vi "Joystick_Test.vi"(9 "input cluster":T7) -> (2 "RobotDriveDevRef":T1={"DevStatus"={"status"=FALSE, "code"=0, "source"=""}, "Motors[]"=[], "Square Inputs"=FALSE, "Max Output"=1.0})   [LabVIEW 2020]
uses:
  <vilib>/Rock Robotics/WPI/RobotDrive/WPI_RobotDriveDevRef.ctl
  <vilib>/Rock Robotics/WPI/MotorControl/WPI_MotorControlDeviceRef.ctl
  <vilib>/Rock Robotics/WPI/MotorControl/WPI_MotorControlType.ctl
  <vilib>/Rock Robotics/SystemInterfaces/DIO/FPGA_DIOPWMChannel.ctl
  <vilib>/Rock Robotics/WPI/PWM/WPI_PWMDeadband.ctl
  <vilib>/Rock Robotics/SystemInterfaces/DIO/FPGA_DIOChannel.ctl
  <vilib>/Rock Robotics/WPI/Utilities/WPI_GetSetVariantRefNum.vi
  <vilib>/Rock Robotics/Network Tables/NT Write Number.vi
  GlobalVariables.vi
  <vilib>/Rock Robotics/WPI/RobotDrive/WPI_RobotDriveArcadeDrive_Standard(NoSaturation).vi
  <vilib>/Rock Robotics/WPI/ThirdParty/Phoenix-LabVIEW/Motor Controller/Controls/CTRE_Phoenix_MotorControl_ControlMode.ctl
panel:
  out "L_X":dbl
  out "L_Y":dbl
  out "Axes[3]":dbl
  out "Axes[2]":dbl
  out "Motor Values":dbl[](array[numeric])
  out "Axes[1]":dbl
  out "Axes[0]":dbl
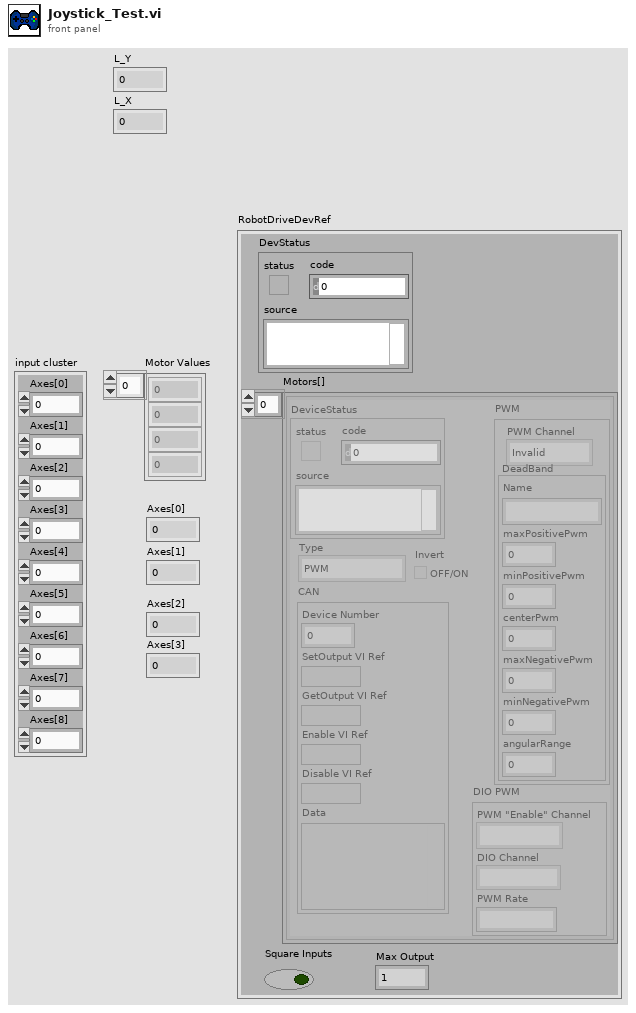
[diagram p1: front panel]
types:
  T1 = typedef "WPI_RobotDriveDevRef.ctl" = cluster{"DevStatus":errorcluster, "Motors[]":T2[], "Square Inputs":bool, "Max Output":dbl}
  T2 = typedef "WPI_MotorControlDeviceRef.ctl" = cluster{"DeviceStatus":errorcluster, "Type":T3, "PWM":cluster{"PWM Channel":T4, "DeadBand":T5}, "CAN":cluster{"Device Number":u8, "SetOutput VI Ref":variant, "GetOutput VI Ref":variant, "Enable VI Ref":variant, "Disable VI Ref":variant, "Data":variant}, "Invert":bool, "DIO PWM":cluster{"PWM \"Enable\" Channel":T4, "DIOChannel":T6, "PWM Rate":dbl}}
  T3 = typedef "WPI_MotorControlType.ctl" = enum16{"PWM", "CAN", "DIO PWM"}
  T4 = typedef "FPGA_DIOPWMChannel.ctl" = enum8{"PWM 0", "PWM 1", "PWM 2", "PWM 3", "PWM 4", "PWM 5", "PWM 6", "PWM 7", "PWM 8", "PWM 9", "PWM MXP 0", "PWM MXP 1", "PWM MXP 2", "PWM MXP 3", "PWM MXP 4", "PWM MXP 5", "PWM MXP 6", "PWM MXP 7", "PWM MXP 8", "PWM MXP 9", "Invalid"}
  T5 = typedef "WPI_PWMDeadband.ctl" = cluster{"Name":string, "maxPositivePwm":i32, "minPositivePwm":i32, "centerPwm":i32, "maxNegativePwm":i32, "minNegativePwm":i32, "angularRange":u16}
  T6 = typedef "FPGA_DIOChannel.ctl" = enum8{"DIO 0", "DIO 1", "DIO 2", "DIO 3", "DIO 4", "DIO 5", "DIO 6", "DIO 7", "DIO 8", "DIO 9", "DIO MXP 0", "DIO MXP 1", "DIO MXP 2", "DIO MXP 3", "DIO MXP 4", "DIO MXP 5", "DIO MXP 6", "DIO MXP 7", "DIO MXP 8", "DIO MXP 9", "DIO MXP 10", "DIO MXP 11", "DIO MXP 12", "DIO MXP 13", "DIO MXP 14", "DIO MXP 15", "SPI Port CS1", "SPI Port CS2", "SPI Port CS3", "SPI Port MISO", "SPI Port MOSI", "Invalid"}
  T7 = cluster{"Axes[0]":dbl, "Axes[1]":dbl, "Axes[2]":dbl, "Axes[3]":dbl, "Axes[4]":dbl, "Axes[5]":dbl, "Axes[6]":dbl, "Axes[7]":dbl, "Axes[8]":dbl}
  T8 = typedef "CTRE_Phoenix_MotorControl_ControlMode.ctl" = u16
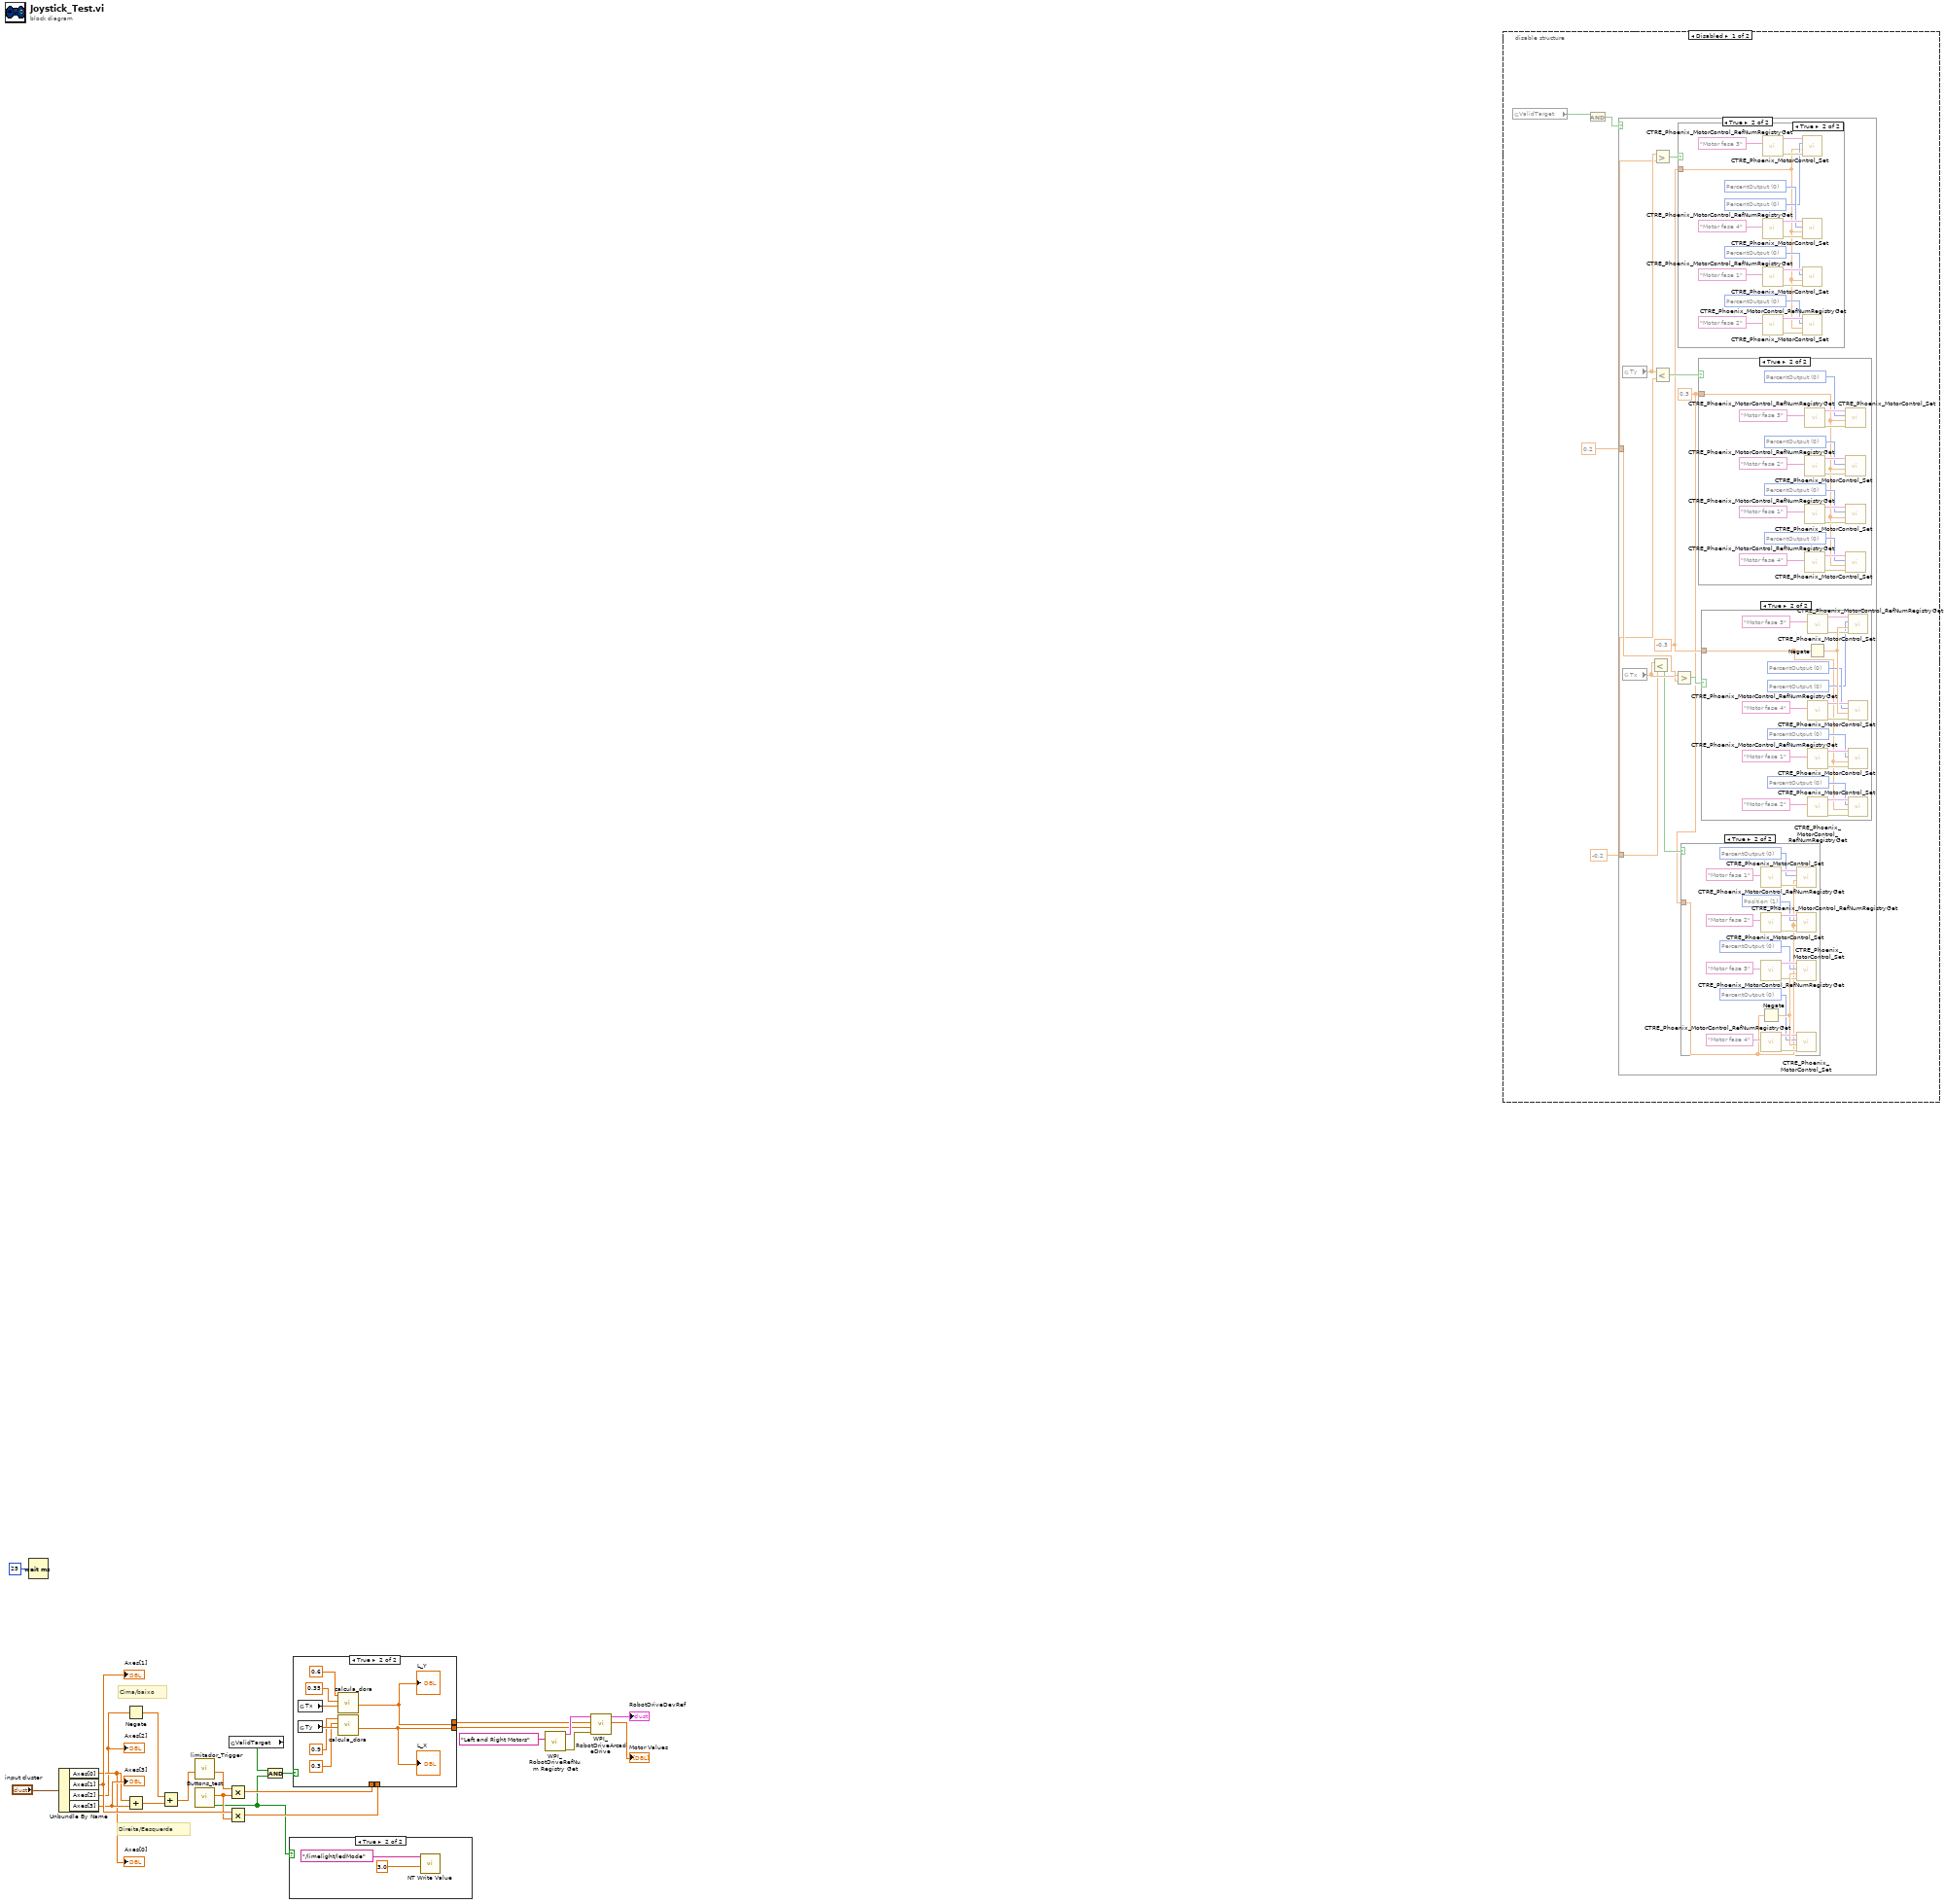
[diagram p0: block diagram]
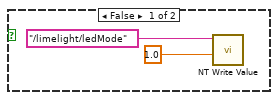
[diagram p2: hidden frame]
diagram:
  # "Direita/Eesquerda"
  # "Cima/baixo"
  n1 = Wait (ms)(milliseconds to wait=u32 25) -> ()  [unwired: 1 out]
  n2 = Unbundle By Name("input cluster") -> ("Axes[0]"=w19:dbl, "Axes[1]"=w23:dbl, "Axes[2]"=w16:dbl, "Axes[3]"=w21:dbl)
  "Axes[0]" <- w19
  "Axes[1]" <- w23
  "Axes[2]" <- w16
  "Axes[3]" <- w21
  n3 = Negate(x=w16) -> (-x=w15:dbl)
  n4 = Add(x=w19, y=w21) -> (x+y=w20:dbl)
  n5 = Add(x=w15, y=w20) -> (x+y=w18:dbl)
  n6 = call "limitador_Trigger.vi"("IN"=w18) -> ("OUT"=w17:dbl)  [unwired: 10 in]
  n7 = call "Buttons_test.vi"() -> ("Buttons[6]"=w1:bool, "OUT"=w22:dbl)  [unwired: 8 in]
  n8 = Multiply(x=w17, y=w22) -> (x*y=w4:dbl)
  n9 = Multiply(x=w23, y=w22) -> (x*y=w5:dbl)
  n10 = global read "GlobalVariables.vi" "ValidTarget"() -> (w11:bool)
  n11 = And(x=w11, y=w1) -> (x .and. y?=w12:bool)
  n12 = case shown="True" w1 {
    frame False {
      n13 = call-poly <vilib>:"NT Write Value.vi"("Numeric"=1.0, "Name"="/limelight/ledMode") -> ()  [unwired: 9 in, 1 out]
    }
    frame True {
      n14 = call-poly <vilib>:"NT Write Value.vi"("Numeric"=3.0, "Name"="/limelight/ledMode") -> ()  [unwired: 9 in, 1 out]
    }
  }
  n15 = case shown="True" w12 {
    tunnel: w5 -> [w29 _]
    tunnel: w4 -> [w28 _]
    tunnel: [w29 w34] -> w3
    tunnel: [w28 w37] -> w2
    frame False {
    }
    frame True {
      n16 = global read "GlobalVariables.vi" "Tx"() -> (w36:dbl)
      n17 = global read "GlobalVariables.vi" "Ty"() -> (w35:dbl)
      n18 = call "calcula_dora.vi"("x"=w36, "Mot_Min"=0.35, "Mot_Max"=0.6) -> ("x+y"=w37:dbl)  [unwired: 8 in]
      "L_Y" <- w37
      n19 = call "calcula_dora.vi"("x"=w35, "Mot_Min"=0.3, "Mot_Max"=0.9) -> ("x+y"=w34:dbl)  [unwired: 8 in]
      "L_X" <- w34
    }
  }
  n20 = call <vilib>:"WPI_RobotDriveRefNum Registry Get.vi"("refnum name"="Left and Right Motors") -> ("error out"=w7:errorcluster, "RobotDriveDevRef"=w9:T1)  [unwired: 9 in]
  n21 = call-poly <vilib>:"WPI_RobotDriveArcadeDrive.vi"("error in (no error)"=w7, "Y axis value"=w3, "X axis value"=w2, "RobotDriveDevRef"=w9) -> ("Motor Values"=→"Motor Values":dbl[], "RobotDriveDevRef"=→"RobotDriveDevRef":T1)  [unwired: 5 in, 1 out]
  n22 = disable-structure shown="Disabled" {
    frame Disabled {
      n23 = global read "GlobalVariables.vi" "ValidTarget"() -> (w41:bool)
      n24 = And(x=w41) -> (x .and. y?=w40:bool)  [unwired: 1 in]
      n25 = case shown="True" w40 {
        tunnel: 0.2 -> [_ w45]
        tunnel: -0.2 -> [_ w44]
        frame False {
        }
        frame True {
          w42 = 0.3
          w43 = -0.3
          n26 = global read "GlobalVariables.vi" "Ty"() -> (w47:dbl)
          n27 = global read "GlobalVariables.vi" "Tx"() -> (w50:dbl)
          n28 = Less?(x=w50, y=w44) -> (x < y?=w49:bool)
          n29 = Greater?(x=w47, y=w45) -> (0:w48:bool)
          n30 = Less?(x=w47, y=w44) -> (x < y?=w46:bool)
          n31 = Greater?(x=w50, y=w45) -> (0:w51:bool)
          n32 = case shown="True" w48 {
            tunnel: w43 -> [_ w69]
            frame False {
            }
            frame True {
              w77 = T8 0 items=["PercentOutput"=0, "Position"=1, "Velocity"=2, "Current"=3, "Follower"=5, "MotionProfile"=6, "MotionMagic"=7, "MotionProfileArc"=10, "Disabled"=15] ("Control Mode")
              w75 = T8 0 items=["PercentOutput"=0, "Position"=1, "Velocity"=2, "Current"=3, "Follower"=5, "MotionProfile"=6, "MotionMagic"=7, "MotionProfileArc"=10, "Disabled"=15] ("Control Mode")
              w73 = T8 0 items=["PercentOutput"=0, "Position"=1, "Velocity"=2, "Current"=3, "Follower"=5, "MotionProfile"=6, "MotionMagic"=7, "MotionProfileArc"=10, "Disabled"=15] ("Control Mode")
              w71 = T8 0 items=["PercentOutput"=0, "Position"=1, "Velocity"=2, "Current"=3, "Follower"=5, "MotionProfile"=6, "MotionMagic"=7, "MotionProfileArc"=10, "Disabled"=15] ("Control Mode")
              n33 = call <vilib>:"CTRE_Phoenix_MotorControl_RefNumRegistryGet.vi"("refnum name"="Motor fase 3") -> ("error out"=w79:errorcluster, "PhoenixMotorControlDevRef"=w78:T2)  [unwired: 9 in]
              n34 = call <vilib>:"CTRE_Phoenix_MotorControl_RefNumRegistryGet.vi"("refnum name"="Motor fase 4") -> ("error out"=w81:errorcluster, "PhoenixMotorControlDevRef"=w80:T2)  [unwired: 9 in]
              n35 = call <vilib>:"CTRE_Phoenix_MotorControl_RefNumRegistryGet.vi"("refnum name"="Motor fase 1") -> ("error out"=w83:errorcluster, "PhoenixMotorControlDevRef"=w82:T2)  [unwired: 9 in]
              n36 = call <vilib>:"CTRE_Phoenix_MotorControl_RefNumRegistryGet.vi"("refnum name"="Motor fase 2") -> ("error out"=w85:errorcluster, "PhoenixMotorControlDevRef"=w84:T2)  [unwired: 9 in]
              n37 = call <vilib>:"CTRE_Phoenix_MotorControl_Set.vi"("error in (no error)"=w79, "Output"=w69, "Control Mode"=w71, "PhoenixMotorControlDevRef"=w78) -> ()  [unwired: 6 in, 2 out]
              n38 = call <vilib>:"CTRE_Phoenix_MotorControl_Set.vi"("error in (no error)"=w81, "Output"=w69, "Control Mode"=w73, "PhoenixMotorControlDevRef"=w80) -> ()  [unwired: 6 in, 2 out]
              n39 = call <vilib>:"CTRE_Phoenix_MotorControl_Set.vi"("error in (no error)"=w83, "Output"=w69, "Control Mode"=w75, "PhoenixMotorControlDevRef"=w82) -> ()  [unwired: 6 in, 2 out]
              n40 = call <vilib>:"CTRE_Phoenix_MotorControl_Set.vi"("error in (no error)"=w85, "Output"=w69, "Control Mode"=w77, "PhoenixMotorControlDevRef"=w84) -> ()  [unwired: 6 in, 2 out]
            }
          }
          n41 = case shown="True" w49 {
            tunnel: w42 -> [_ w86]
            frame False {
            }
            frame True {
              w94 = T8 0 items=["PercentOutput"=0, "Position"=1, "Velocity"=2, "Current"=3, "Follower"=5, "MotionProfile"=6, "MotionMagic"=7, "MotionProfileArc"=10, "Disabled"=15] ("Control Mode")
              w92 = T8 0 items=["PercentOutput"=0, "Position"=1, "Velocity"=2, "Current"=3, "Follower"=5, "MotionProfile"=6, "MotionMagic"=7, "MotionProfileArc"=10, "Disabled"=15] ("Control Mode")
              w90 = T8 1 items=["PercentOutput"=0, "Position"=1, "Velocity"=2, "Current"=3, "Follower"=5, "MotionProfile"=6, "MotionMagic"=7, "MotionProfileArc"=10, "Disabled"=15] ("Control Mode")
              w88 = T8 0 items=["PercentOutput"=0, "Position"=1, "Velocity"=2, "Current"=3, "Follower"=5, "MotionProfile"=6, "MotionMagic"=7, "MotionProfileArc"=10, "Disabled"=15] ("Control Mode")
              n42 = call <vilib>:"CTRE_Phoenix_MotorControl_RefNumRegistryGet.vi"("refnum name"="Motor fase 1") -> ("error out"=w96:errorcluster, "PhoenixMotorControlDevRef"=w95:T2)  [unwired: 9 in]
              n43 = call <vilib>:"CTRE_Phoenix_MotorControl_RefNumRegistryGet.vi"("refnum name"="Motor fase 2") -> ("error out"=w98:errorcluster, "PhoenixMotorControlDevRef"=w97:T2)  [unwired: 9 in]
              n44 = call <vilib>:"CTRE_Phoenix_MotorControl_RefNumRegistryGet.vi"("refnum name"="Motor fase 3") -> ("error out"=w100:errorcluster, "PhoenixMotorControlDevRef"=w99:T2)  [unwired: 9 in]
              n45 = Negate(x=w86) -> (-x=w103:dbl)
              n46 = call <vilib>:"CTRE_Phoenix_MotorControl_RefNumRegistryGet.vi"("refnum name"="Motor fase 4") -> ("error out"=w102:errorcluster, "PhoenixMotorControlDevRef"=w101:T2)  [unwired: 9 in]
              n47 = call <vilib>:"CTRE_Phoenix_MotorControl_Set.vi"("error in (no error)"=w96, "Output"=w86, "Control Mode"=w88, "PhoenixMotorControlDevRef"=w95) -> ()  [unwired: 6 in, 2 out]
              n48 = call <vilib>:"CTRE_Phoenix_MotorControl_Set.vi"("error in (no error)"=w98, "Output"=w86, "Control Mode"=w90, "PhoenixMotorControlDevRef"=w97) -> ()  [unwired: 6 in, 2 out]
              n49 = call <vilib>:"CTRE_Phoenix_MotorControl_Set.vi"("error in (no error)"=w100, "Output"=w103, "Control Mode"=w92, "PhoenixMotorControlDevRef"=w99) -> ()  [unwired: 6 in, 2 out]
              n50 = call <vilib>:"CTRE_Phoenix_MotorControl_Set.vi"("error in (no error)"=w102, "Output"=w103, "Control Mode"=w94, "PhoenixMotorControlDevRef"=w101) -> ()  [unwired: 6 in, 2 out]
            }
          }
          n51 = case shown="True" w46 {
            tunnel: w42 -> [_ w52]
            frame False {
            }
            frame True {
              w60 = T8 0 items=["PercentOutput"=0, "Position"=1, "Velocity"=2, "Current"=3, "Follower"=5, "MotionProfile"=6, "MotionMagic"=7, "MotionProfileArc"=10, "Disabled"=15] ("Control Mode")
              w58 = T8 0 items=["PercentOutput"=0, "Position"=1, "Velocity"=2, "Current"=3, "Follower"=5, "MotionProfile"=6, "MotionMagic"=7, "MotionProfileArc"=10, "Disabled"=15] ("Control Mode")
              w56 = T8 0 items=["PercentOutput"=0, "Position"=1, "Velocity"=2, "Current"=3, "Follower"=5, "MotionProfile"=6, "MotionMagic"=7, "MotionProfileArc"=10, "Disabled"=15] ("Control Mode")
              w54 = T8 0 items=["PercentOutput"=0, "Position"=1, "Velocity"=2, "Current"=3, "Follower"=5, "MotionProfile"=6, "MotionMagic"=7, "MotionProfileArc"=10, "Disabled"=15] ("Control Mode")
              n52 = call <vilib>:"CTRE_Phoenix_MotorControl_RefNumRegistryGet.vi"("refnum name"="Motor fase 3") -> ("error out"=w62:errorcluster, "PhoenixMotorControlDevRef"=w61:T2)  [unwired: 9 in]
              n53 = call <vilib>:"CTRE_Phoenix_MotorControl_RefNumRegistryGet.vi"("refnum name"="Motor fase 2") -> ("error out"=w68:errorcluster, "PhoenixMotorControlDevRef"=w67:T2)  [unwired: 9 in]
              n54 = call <vilib>:"CTRE_Phoenix_MotorControl_RefNumRegistryGet.vi"("refnum name"="Motor fase 1") -> ("error out"=w66:errorcluster, "PhoenixMotorControlDevRef"=w65:T2)  [unwired: 9 in]
              n55 = call <vilib>:"CTRE_Phoenix_MotorControl_RefNumRegistryGet.vi"("refnum name"="Motor fase 4") -> ("error out"=w64:errorcluster, "PhoenixMotorControlDevRef"=w63:T2)  [unwired: 9 in]
              n56 = call <vilib>:"CTRE_Phoenix_MotorControl_Set.vi"("error in (no error)"=w62, "Output"=w52, "Control Mode"=w54, "PhoenixMotorControlDevRef"=w61) -> ()  [unwired: 6 in, 2 out]
              n57 = call <vilib>:"CTRE_Phoenix_MotorControl_Set.vi"("error in (no error)"=w68, "Output"=w52, "Control Mode"=w60, "PhoenixMotorControlDevRef"=w67) -> ()  [unwired: 6 in, 2 out]
              n58 = call <vilib>:"CTRE_Phoenix_MotorControl_Set.vi"("error in (no error)"=w66, "Output"=w52, "Control Mode"=w58, "PhoenixMotorControlDevRef"=w65) -> ()  [unwired: 6 in, 2 out]
              n59 = call <vilib>:"CTRE_Phoenix_MotorControl_Set.vi"("error in (no error)"=w64, "Output"=w52, "Control Mode"=w56, "PhoenixMotorControlDevRef"=w63) -> ()  [unwired: 6 in, 2 out]
            }
          }
          n60 = case shown="True" w51 {
            tunnel: w43 -> [_ w104]
            frame False {
            }
            frame True {
              w112 = T8 0 items=["PercentOutput"=0, "Position"=1, "Velocity"=2, "Current"=3, "Follower"=5, "MotionProfile"=6, "MotionMagic"=7, "MotionProfileArc"=10, "Disabled"=15] ("Control Mode")
              w110 = T8 0 items=["PercentOutput"=0, "Position"=1, "Velocity"=2, "Current"=3, "Follower"=5, "MotionProfile"=6, "MotionMagic"=7, "MotionProfileArc"=10, "Disabled"=15] ("Control Mode")
              w108 = T8 0 items=["PercentOutput"=0, "Position"=1, "Velocity"=2, "Current"=3, "Follower"=5, "MotionProfile"=6, "MotionMagic"=7, "MotionProfileArc"=10, "Disabled"=15] ("Control Mode")
              w106 = T8 0 items=["PercentOutput"=0, "Position"=1, "Velocity"=2, "Current"=3, "Follower"=5, "MotionProfile"=6, "MotionMagic"=7, "MotionProfileArc"=10, "Disabled"=15] ("Control Mode")
              n61 = call <vilib>:"CTRE_Phoenix_MotorControl_RefNumRegistryGet.vi"("refnum name"="Motor fase 3") -> ("error out"=w118:errorcluster, "PhoenixMotorControlDevRef"=w117:T2)  [unwired: 9 in]
              n62 = Negate(x=w104) -> (-x=w121:dbl)
              n63 = call <vilib>:"CTRE_Phoenix_MotorControl_RefNumRegistryGet.vi"("refnum name"="Motor fase 4") -> ("error out"=w120:errorcluster, "PhoenixMotorControlDevRef"=w119:T2)  [unwired: 9 in]
              n64 = call <vilib>:"CTRE_Phoenix_MotorControl_RefNumRegistryGet.vi"("refnum name"="Motor fase 1") -> ("error out"=w114:errorcluster, "PhoenixMotorControlDevRef"=w113:T2)  [unwired: 9 in]
              n65 = call <vilib>:"CTRE_Phoenix_MotorControl_RefNumRegistryGet.vi"("refnum name"="Motor fase 2") -> ("error out"=w116:errorcluster, "PhoenixMotorControlDevRef"=w115:T2)  [unwired: 9 in]
              n66 = call <vilib>:"CTRE_Phoenix_MotorControl_Set.vi"("error in (no error)"=w118, "Output"=w121, "Control Mode"=w110, "PhoenixMotorControlDevRef"=w117) -> ()  [unwired: 6 in, 2 out]
              n67 = call <vilib>:"CTRE_Phoenix_MotorControl_Set.vi"("error in (no error)"=w120, "Output"=w121, "Control Mode"=w112, "PhoenixMotorControlDevRef"=w119) -> ()  [unwired: 6 in, 2 out]
              n68 = call <vilib>:"CTRE_Phoenix_MotorControl_Set.vi"("error in (no error)"=w114, "Output"=w104, "Control Mode"=w106, "PhoenixMotorControlDevRef"=w113) -> ()  [unwired: 6 in, 2 out]
              n69 = call <vilib>:"CTRE_Phoenix_MotorControl_Set.vi"("error in (no error)"=w116, "Output"=w104, "Control Mode"=w108, "PhoenixMotorControlDevRef"=w115) -> ()  [unwired: 6 in, 2 out]
            }
          }
        }
      }
    }
    frame Enabled {
    }
  }
